vi "Create Plots(SubVI).vi"(11 "NavData Out":T1) -> (1 "Numeric 2":sgl, 2 "yaw (deg)":sgl, 3 "altitude (cm)":u32, 4 "Numeric":sgl)   [LabVIEW 2014]
uses:
  <vilib>/LVH/AR Drone Toolkit/Decode NavData/Typedefs/NavData Demo.ctl
  <vilib>/LVH/AR Drone Toolkit/AR Drone.lvlib
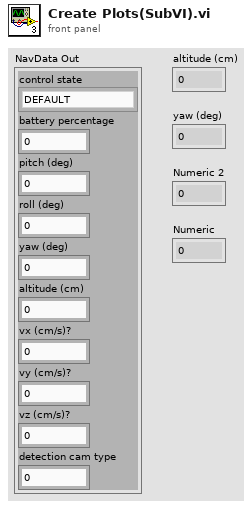
[diagram p1: front panel]
types:
  T1 = typedef "AR Drone.lvlib/NavData Demo.ctl" = cluster{"control state":enum32{"DEFAULT", "INIT", "LANDING", "FLYING", "HOVERING", "TEST", "TRANS_TAKEOFF", "TRANS_GOTOFIX", "TRANS_LANDING"}, "battery percentage":u32, "pitch (deg)":sgl, "roll (deg)":sgl, "yaw (deg)":sgl, "altitude (cm)":u32, "vx (cm/s)?":sgl, "vy (cm/s)?":sgl, "vz (cm/s)?":sgl, "detection cam type":u32}
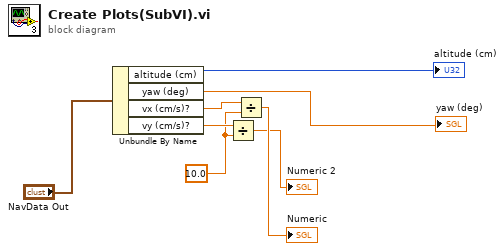
[diagram p0: block diagram]
diagram:
  w1 = sgl 10.0 ("y")
  n1 = Unbundle By Name("NavData Out") -> ("altitude (cm)"=→"altitude (cm)":u32, "yaw (deg)"=→"yaw (deg)":sgl, "vx (cm/s)?"=w4:sgl, "vy (cm/s)?"=w5:sgl)
  n2 = Divide(x=w5, y=w1) -> (x/y=→"Numeric 2":sgl)
  n3 = Divide(x=w4, y=w1) -> (x/y=→"Numeric":sgl)
